vi "Write Local Error.vi"(8 "error in (no error)":errorcluster, 11 "CIF_UI in":refnum<class "CIF_UI.lvclass">) -> (0 "error out":errorcluster)   [LabVIEW 2021, in "CIF_UI.lvclass"]
doc: "Provide a human readable error message to the local error display from the calling VI. This is used when a subpanel is created for the plugin. This allows any errors to be passed to the error display."
uses:
  CIF_UI.lvclass
  CIF_UI.lvclass/CIF_UI.ctl
  <vilib>/CIF Foundation/CIF Utilities/Errors/Human Readable Error Message.vi
  <vilib>/CIF Foundation/CIF Utilities/Errors/Errors_CIF_U.lvlib
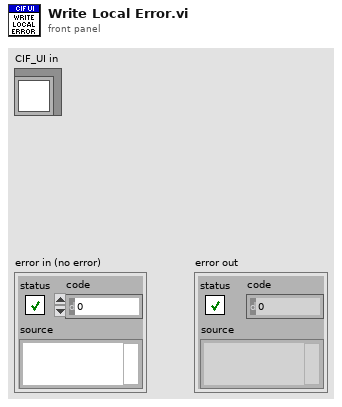
[diagram p1: front panel]
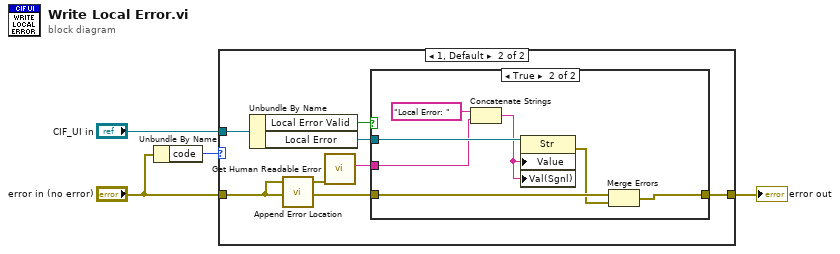
[diagram p0: block diagram]
diagram:
  n1 = Unbundle By Name("error in (no error)") -> ("code"=w1:i32)
  n2 = case shown="1, Default" w1 {
    tunnel: "CIF_UI in" -> [_ w12]
    tunnel: [w5 w9] -> w3
    tunnel: "error in (no error)" -> [w5 w7]
    frame 0 {
    }
    frame 1, Default {
      n3 = Unbundle By Name(w12) -> ("Local Error Valid"=w11:bool, "Local Error"=w10:refnum<vi>)
      n4 = call <vilib>:"Append Error Location.vi"("error in (no error)"=w7) -> ("error out"=w6:errorcluster)  [unwired: 4 in]
      n5 = call "Get Human Readable Error.vi"("error in (no error)"=w6) -> ("Error Message"=w8:string)  [unwired: 10 in]
      n6 = case shown="True" w11 {
        tunnel: w10 -> [_ w20]
        tunnel: w8 -> [_ w18]
        tunnel: w7 -> [w13 w16]
        tunnel: [w13 w14] -> w9
        frame False {
        }
        frame True {
          n7 = Concatenate Strings("Local Error: " ("string"), w18) -> (w17:string)
          n8 = property class="Str"(reference=w20, "Value"=w17, "Val(Sgnl)"=w17) -> (error out=w15:errorcluster)  [unwired: 1 in, 1 out]
          n9 = Merge Errors(w16, w15) -> (w14:errorcluster)
        }
      }
    }
  }
  "error out" <- w3
